vi "Kill Em All.vi"() -> ()   [LabVIEW 2018]
uses:
  <resource>/objmgr/daqmx.rc
panel:
  out "Tasks":refnum<k21>[](array[refnum])
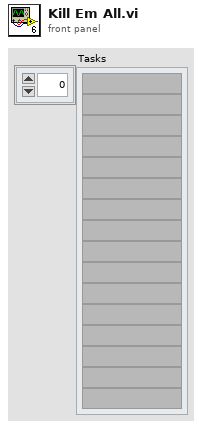
[diagram p1: front panel]
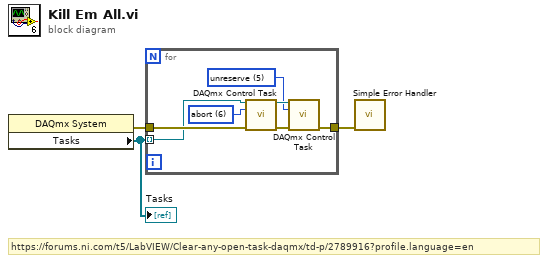
[diagram p0: block diagram]
diagram:
  # "https://forums.ni.com/t5/LabVIEW/Clear-any-open-task-daqmx/td-p/2789916?profile.language=en"
  n1 = property class="DAQmx System"() -> (error out=w2:errorcluster, "Tasks"=w3:refnum<k21>[])  [unwired: 2 in, 1 out]
  "Tasks" <- w3
  n2 = for {
    tunnel: w3 -> [w7] mode=indexing
    tunnel: w2 -> [w8]
    tunnel: [w4] -> w1
    w5 = 5 items=["verify"=2, "reserve"=4, "commit"=3, "unreserve"=5, "abort"=6] ("action")
    w6 = 6 items=["verify"=2, "reserve"=4, "commit"=3, "unreserve"=5, "abort"=6] ("action")
    n3 = call <vilib>:"DAQmx Control Task.vi"("task/channels in"=w7, "action"=w6, "error in"=w8) -> ("task out"=w9:refnum<k21>, "error out"=w10:errorcluster)  [unwired: 11 in]
    n4 = call <vilib>:"DAQmx Control Task.vi"("task/channels in"=w9, "action"=w5, "error in"=w10) -> ("error out"=w4:errorcluster)  [unwired: 11 in, 1 out]
  }
  n5 = call <vilib>:"Simple Error Handler.vi"("error in (no error)"=w1) -> ()  [unwired: 4 in, 5 out]
